vi "Subtraction.vi"(9 "y":dbl, 10 "x":dbl) -> (2 "x-y":dbl)   [LabVIEW 2018]
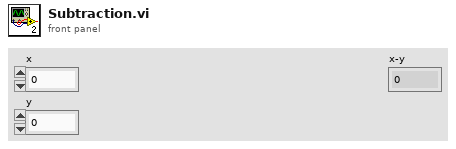
[diagram p1: front panel]
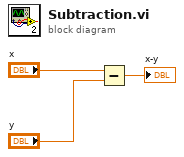
[diagram p0: block diagram]
diagram:
  n1 = Subtract(x="x", y="y") -> (x-y=→"x-y":dbl)
